vi "Array Size(s).vi"(8 "错误输入":errorcluster, 10 "Array":variant) -> (0 "错误输出":errorcluster, 1 "N dims":u32, 2 "Size(s)":u32[](array[numeric]))   [LabVIEW 2012, in "TD Tools.lvlib"]
uses:
  TD Tools.lvlib
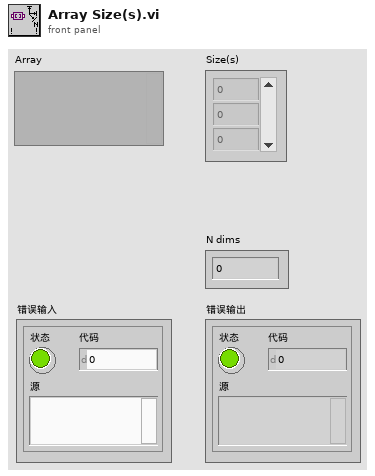
[diagram p1: front panel]
types:
  T1 = typedef "TD Tools.lvlib/Type Descriptor Header.ctl" = cluster{"length":u16, "private":u8, "type":T2, "# elements":u16}
  T2 = typedef "TD Tools.lvlib/Type Descriptor Enumeration.ctl" = enum16{"<Null>", "I8", "I16", "I32", "I64", "U8", "U16", "U32", "U64", "SGL", "DBL", "EXT", "CSG", "CDB", "CXT", "0x0F", "0x10", "0x11", "0x12", "0x13", "0x14", "Enum U8", "Enum U16", "Enum U32", "Enum U64", "SGL PQ", "DBL PQ", "EXT PQ", "CSG PQ", "CDB PQ", "CXT PQ", "0x1F", "0x20", "Boolean", "0x22", "0x23", "0x24", "0x25", "0x26", "0x27", "0x28", "0x29", "0x2A", "0x2B", "0x2C", "0x2D", "0x2E", "0x2F", "String", "0x31", "Path", "Pict", "0x34", "0x35", "0x36", "DAQ", "0x38", "0x39", "0x3A", "0x3B", "0x3C", "0x3D", "0x3E", "0x3F", "Array", "0x41", "0x42", "0x43", "0x44", "0x45", "0x46", "0x47", "0x48", "0x49", "0x4A", "0x4B", "0x4C", "0x4D", "0x4E", "0x4F", "Cluster", "0x51", "0x52", "Variant", "Waveform", "0x55", "0x56", "0x57", "0x58", "0x59", "0x5A", "0x5B", "0x5C", "0x5D", "0x5E", "0x5F", "0x60", "0x61", "0x62", "0x63", "0x64", "0x65", "0x66", "0x67", "0x68", "0x69", "0x6A", "0x6B", "0x6C", "0x6D", "0x6E", "0x6F", "Refnum"}
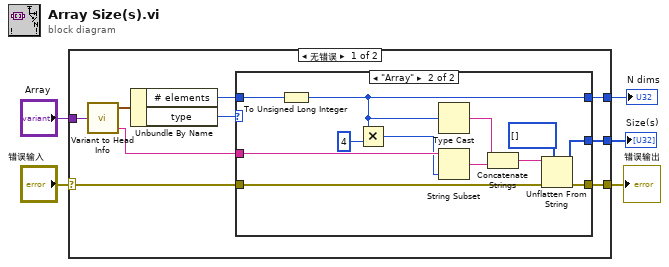
[diagram p0: block diagram]
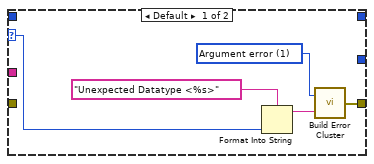
[diagram p2: hidden frame]
diagram:
  n1 = case shown="无错误" "错误输入" {
    selector: "错误输入" -> [w6 w32]
    tunnel: [w11 w32] -> w4
    tunnel: "Array" -> [w14 _]
    tunnel: [w9 _] -> w2
    tunnel: [w7 _] -> w1
    frame No Error {
      n2 = call "Variant to Head Info.vi"("Variant"=w14) -> ("Data String"=w8:string, "Type Descriptor Header"=w13:T1)  [unwired: 2 in, 1 out]
      n3 = Unbundle By Name(w13) -> ("# elements"=w10:u16, "type"=w12:T2)
      n4 = case shown="\"Array\"" w12 {
        selector: w12 -> [w19 _]
        tunnel: [w15 w20] -> w11
        tunnel: w10 -> [_ w31]
        tunnel: [_ w27] -> w9
        tunnel: w8 -> [_ w29]
        tunnel: [_ w22] -> w7
        tunnel: w6 -> [_ w21]
        frame Default {
          w17 = 1 items=["No error", "Argument error", "Memory is full", "Out of zone", "End of file", "File already open", "Generic file I/O error", "File not found", "File permission error", "Disk is full", "Duplicate path", "Too many files open", "System feature not enabled", "Resource file not found", "Cannot add resource", "Resource not found", "Image not found", "Image memory error", "Pen does not exist", "Config type invalid", "Config token not found", "Config parse error", "Config memory error", "Bad external code format", "Bad external code offset", "External code not present", "Null window", "Destroy window error", "Null menu", "Print aborted", "Bad print record", "Print driver error", "Windows error during printing", "Memory error during printing", "Print dialog error", "Generic print error", "Invalid device refnum", "Device not found", "Device parameter error", "Device unit error", "Cannot open device", "Device call aborted", "Generic error", "Cancelled by user", "Object ID too low", "Object ID too high", "Object not in heap", "Unknown heap", "Unknown object (invalid DefProc)", "Unknown object (DefProc not in table)", "Message out of range", "Invalid (null) method", "Unknown message", "Manager call not supported", "Bad address", "Network operation in progress", "Network operation timed out", "Connection is busy", "Network attribute not supported", "Network error", "Address in use", "System out of memory", "Connection aborted", "Connection refused", "Not connected", "Already connected", "Connection closed", "Initialization error (interapplication manager)", "Bad occurrence", "Wait on unbound occurrence handler", "Occurrence queue overflow", "Datalog type conflict", "Unused", "Unrecognized type (interapplication manager)", "Memory corrupt", "Failed to make temporary DLL", "Old CIN version", "Drag socket not found", "Failed to load drop-object", "Failed to register OLE object", "Failed to release OLE object", "Format specifier type mismatch", "Unknown format specifier", "Too few format specifiers", "Too many format specifiers", "Scan failed", "Newer CIN version", "Error converting to variant", "Runtime menu error", "Password tampered", "Variant attribute not found", "Incompatible variant data type", "Event data is not available", "Event Store is not present", "Occurrence is not found", "Event Queue is not created", "Event info is not available", "Refnum passed is NULL", "Error retrieving Class GUID", "Error retrieving CoClass GUID", "Error retrieving TypeLib GUID.", "Bad built application magic bytes.", "Specific driver is different from the specific driver associated with the Logical Name.", "There is no session opened to the class driver.", "Max Error", "MAX - Error with config objects", "MAX - Error loading configuration", "MAX - Group not supported"]
          n5 = Format Into String(format string="Unexpected Datatype <%s>" ("Format String"), w19) -> (resulting string=w16:string)  [unwired: 2 in, 1 out]
          n6 = call "Build Error Cluster.vi"("String to Prepend to source (\"\")"=w16, "code"=w17) -> ("error out"=w15:errorcluster)
        }
        frame "Array" {
          n7 = To Unsigned Long Integer(number=w31) -> (unsigned 32bit integer=w27:u32)
          n8 = Multiply(x=w27, y=u32 4) -> (x*y=w28:u32)
          n9 = Type Cast(x=w27) -> (*(type *) &x=w26:string)  [unwired: 1 in]
          n10 = String Subset(string=w29, length (rest)=w28) -> (substring=w25:string)  [unwired: 1 in]
          n11 = Concatenate Strings(w26, w25) -> (w24:string)
          n12 = Unflatten From String(type=u32[] [] ("Size(s)"), binary string=w24, error in (no error)=w21) -> (value=w22:u32[], error out=w20:errorcluster)  [unwired: 2 in, 1 out]
        }
      }
    }
    frame Error {
    }
  }
  "错误输出" <- w4
  "Size(s)" <- w1
  "N dims" <- w2
